vi "data_process_packet.vi"(6 "Sensor Lookup Indices":i32[](array[numeric]), 7 "Gains":dbl[](array[numeric])=[1.502, 1.502, 2.42], 8 "error in (no error)":errorcluster, 10 "No. Sensors":i32=128, 11 "Binary Input Data":string) -> (0 "error out":errorcluster, 1 "Raw Sensors N x XYZ":dbl[][](array[numeric]), 2 "Raw Sensors (Flattened)":i16[](array[numeric]), 3 "Time":u32, 4 "Sensors (uT)":dbl[][](array[numeric]))   [LabVIEW 2018]
panel:
  out "index of element 2":i32
  in  "threshold 2":dbl
  out "Z data 2":dbl[](graph)
  in  "byte order (0:big-endian, network order)":T1(ring)=enum."little-endian"
  out "Time Packet":string
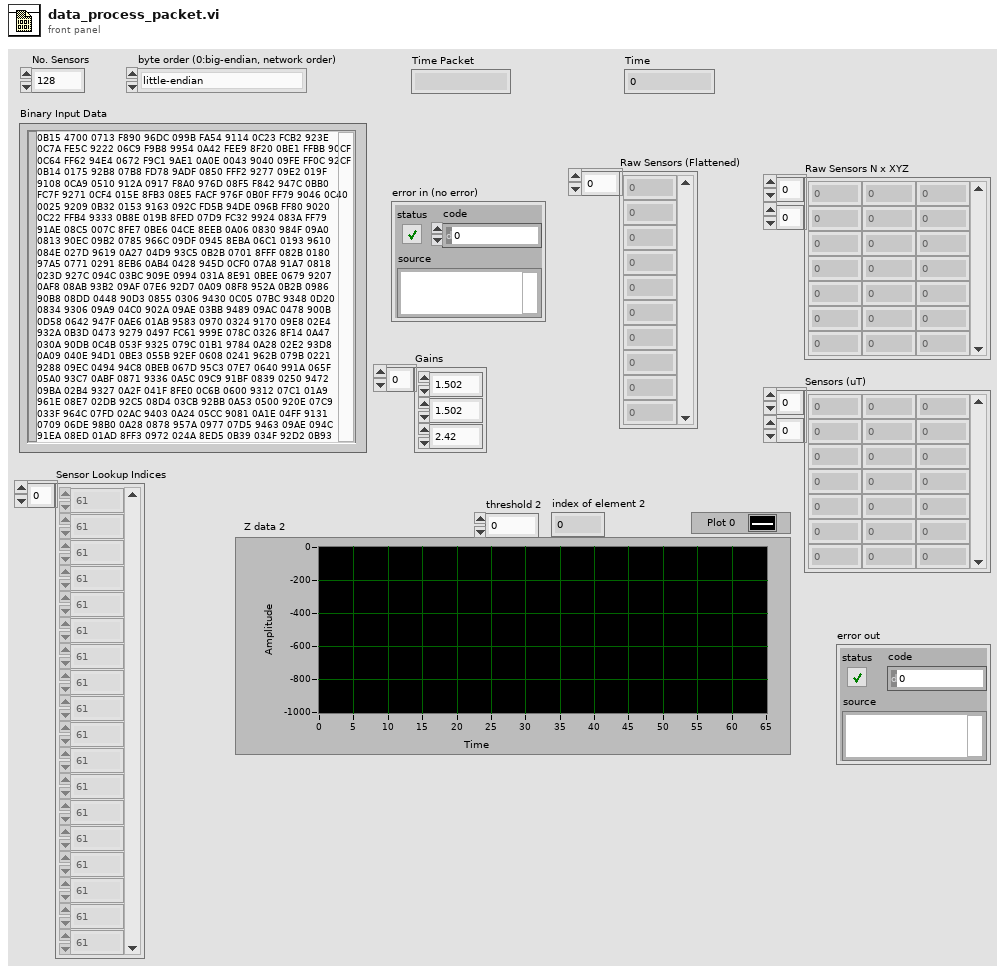
[diagram p1: front panel]
types:
  T1 = enum16{"big-endian, network order", "native, host order", "little-endian"}
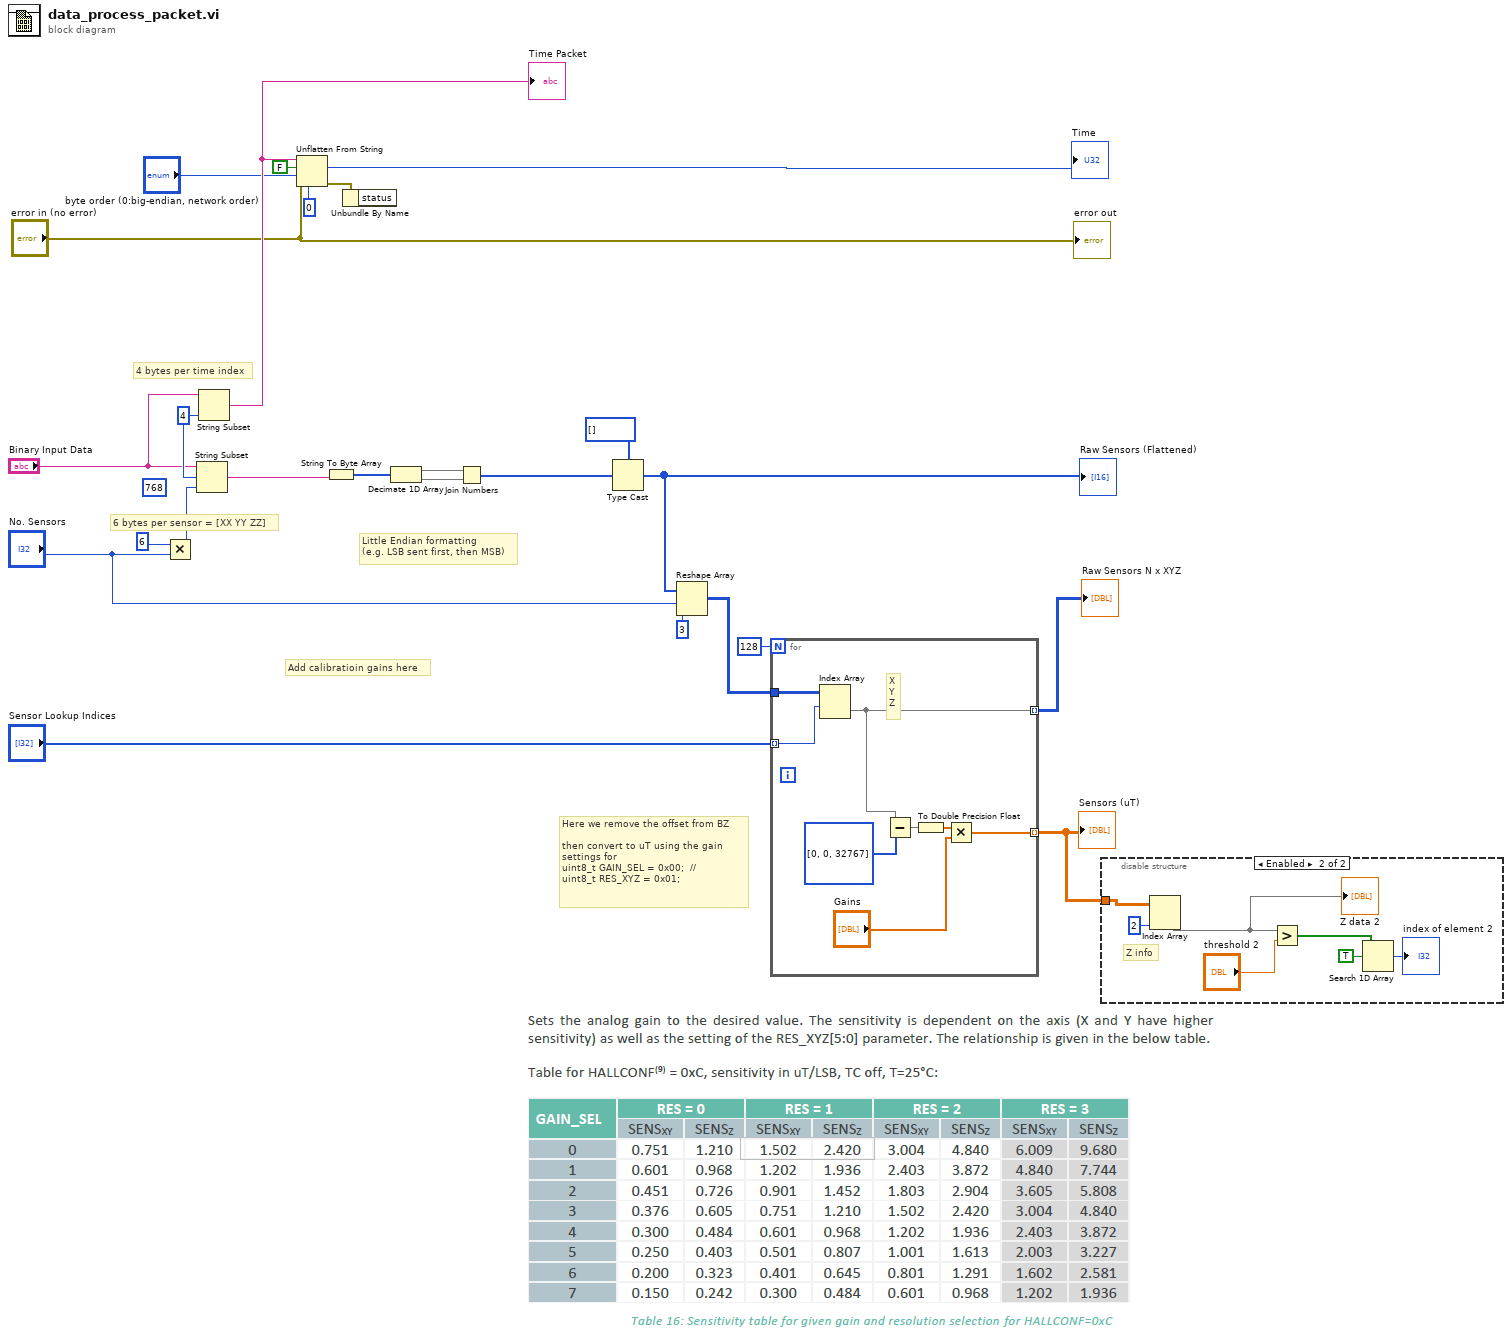
[diagram p0: block diagram]
diagram:
  (unwired) 768 ("length (rest)")
  w25 = 4 ("length (rest)")
  # "Here we remove the offset from BZ\n\nthen convert to uT using the gain\nsettings for \nuint8_t GAIN_SEL = 0x00;  // \nuint8_t RES_XYZ = 0x01;"
  # "Add calibratioin gains here"
  # "4 bytes per time index"
  # "6 bytes per sensor = [XX YY ZZ]"
  # "Little Endian formatting\n(e.g. LSB sent first, then MSB)"
  n1 = Multiply(x=6 ("length (rest)"), y="No. Sensors") -> (x*y=w8:i32)
  n2 = String Subset(string="Binary Input Data", offset (0)=w25, length (rest)=w8) -> (substring=w22:string)
  n3 = String Subset(string="Binary Input Data", length (rest)=w25) -> (substring=w24:string)  [unwired: 1 in]
  "Time Packet" <- w24
  n4 = Unflatten From String(type=u32 0 ("default (0 U32)"), binary string=w24, data includes array or string size? (T)=FALSE, byte order (0:big-endian, network order)="byte order (0:big-endian, network order)", error in (no error)="error in (no error)") -> (value=→"Time":u32, error out=w13:errorcluster)  [unwired: 1 out]
  n5 = String To Byte Array(string=w22) -> (unsigned byte array=w21:u8[])
  n6 = Unbundle By Name(w13) -> ()  [unwired: 1 out]
  n7 = Decimate 1D Array(w21) -> (w18:u8[], w17:u8[])
  n8 = Join Numbers(hi=w18, lo=w17) -> ((hi.lo)=w15:u16[])
  n9 = Type Cast(type=i16[] [], x=w15) -> (*(type *) &x=w7:i16[])
  "Raw Sensors (Flattened)" <- w7
  n10 = Reshape Array(w7, "No. Sensors", 3 ("milliseconds to wait")) -> (w5:i16[][])
  n11 = for {
    N: 128 -> [_]
    tunnel: w5 -> [w33]
    tunnel: [w32] -> w4 mode=indexing
    tunnel: [w27] -> w3 mode=indexing
    tunnel: "Sensor Lookup Indices" -> [w26] mode=indexing
    # "X\nY \nZ"
    n12 = Index Array(array=w33, index (row)=w26) -> (element=w32:i16[])  [unwired: 1 in]
    n13 = Subtract(x=w32, y=i16[] [0, 0, 32767]) -> (x-y=w30:i16[])
    n14 = To Double Precision Float(number=w30) -> (double precision float=w29:dbl[])
    n15 = Multiply(x=w29, y="Gains") -> (x*y=w27:dbl[])
  }
  "Raw Sensors N x XYZ" <- w4
  "Sensors (uT)" <- w3
  n16 = disable-structure shown="Enabled" {
    disable-tunnel: w3 -> [_ w34]
    frame Disabled {
    }
    frame Enabled {
      # "Z info"
      n17 = Index Array(array=w34, index (col)=2 ("disabled index (col)")) -> (element=w38:dbl[])  [unwired: 1 in]
      "Z data 2" <- w38
      n18 = Greater?(x=w38, y="threshold 2") -> (0:w39:bool[])
      n19 = Search 1D Array(1D array=w39, element=TRUE) -> (index of element=→"index of element 2":i32)  [unwired: 1 in]
    }
  }
  "error out" <- "error in (no error)"
